vi "VD_SetVoltage_Increase.vi"(8 "error in (no error)":errorcluster, 9 "Vt [V]":ext=40.0, 10 "Vdc [V]":ext=40.0, 11 "VISA VD_Supply":refnum<visa-resource-name>) -> (0 "error out":errorcluster, 1 "Vt_Array":ext[](array[numeric]), 2 "Vdc_Array":ext[](array[numeric]), 3 "VISA VD_Supply 2":refnum<visa-resource-name>, 4 "Inv_Vt_Array":ext[](array[numeric]), 5 "Inv_Vdc_Array":ext[](array[numeric]))   [LabVIEW 2017]
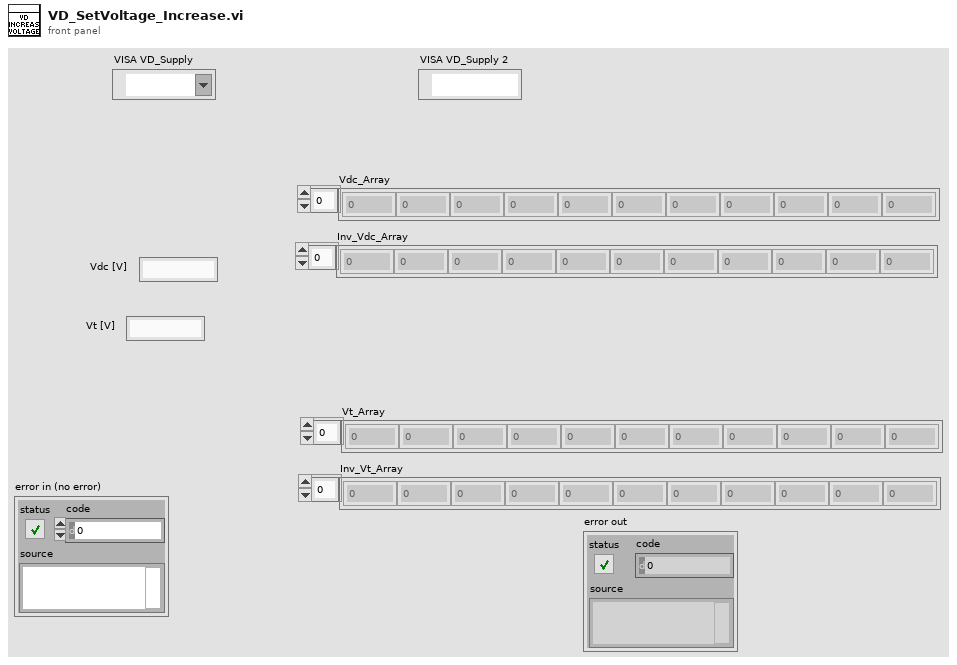
[diagram p1: front panel]
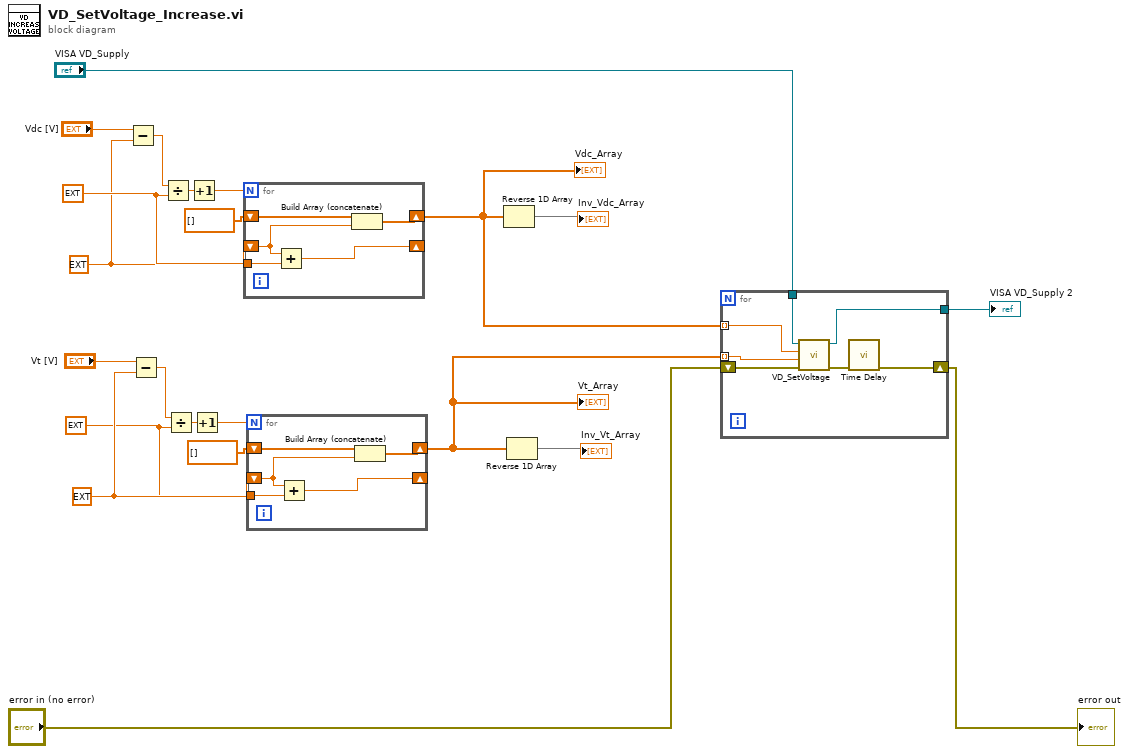
[diagram p0: block diagram]
diagram:
  w12 = ext 0.0 ("Start_freq [Hz]")
  w7 = ext 0.1 ("Step_freq [Hz]")
  w17 = ext 0.0 ("Start_freq [Hz]")
  w22 = ext 0.1 ("Step_freq [Hz]")
  n1 = Subtract(x="Vdc [V]", y=w17) -> (x-y=w16:ext)
  n2 = Subtract(x="Vt [V]", y=w12) -> (x-y=w13:ext)
  n3 = Divide(x=w16, y=w22) -> (x/y=w19:ext)
  n4 = Divide(x=w13, y=w7) -> (x/y=w10:ext)
  n5 = Increment(x=w19) -> (x+1=w20:ext)
  n6 = Increment(x=w10) -> (x+1=w9:ext)
  n7 = for {
    N: w20 -> [_]
    tunnel: w22 -> [w27]
    shift-right: [w25] -> w6
    shift-left: ext[] [] -> [w24]
    shift-right: [w26] -> _
    shift-left: w17 -> [w23]
    n8 = Add(x=w23, y=w27) -> (x+y=w26:ext)
    n9 = Build Array (concatenate)(w24, w23) -> (w25:ext[])
  }
  "Vdc_Array" <- w6
  n10 = for {
    N: w9 -> [_]
    tunnel: w7 -> [w32]
    shift-right: [w30] -> w5
    shift-left: ext[] [] -> [w29]
    shift-right: [w31] -> _
    shift-left: w12 -> [w28]
    n11 = Add(x=w28, y=w32) -> (x+y=w31:ext)
    n12 = Build Array (concatenate)(w29, w28) -> (w30:ext[])
  }
  "Vt_Array" <- w5
  n13 = Reverse 1D Array(array=w6) -> (reversed array=→"Inv_Vdc_Array":ext[])
  n14 = Reverse 1D Array(array=w5) -> (reversed array=→"Inv_Vt_Array":ext[])
  n15 = for {
    tunnel: w6 -> [w39] mode=indexing
    shift-right: [w37] -> w2
    shift-left: "error in (no error)" -> [w36]
    tunnel: w5 -> [w35] mode=indexing
    tunnel: "VISA VD_Supply" -> [w34]
    tunnel: [w33] -> w3
    n16 = call "VD_SetVoltage.vi"("error in"=w36, "Vout2"=w35, "Vout1"=w39, "VISA VD_Supply"=w34) -> ("error out"=w38:errorcluster, "VISA VD_Supply"=w33:refnum<visa-resource-name>)  [unwired: 6 in]
    n17 = call "Time Delay"("error in (no error)"=w38) -> ("error out"=w37:errorcluster)  [unwired: 10 in]
  }
  "error out" <- w2
  "VISA VD_Supply 2" <- w3
